vi "Get KeyValues.vi"(8 "error in (no error)":errorcluster, 11 "Frames":refnum<k21>[](array[refnum])) -> (0 "error out":errorcluster, 1 "<JSON>":string caption="<JSON>Object", 2 "Sigs":refnum<k21>[](array[refnum]), 3 "Signal Names":string[](array[string]))   [LabVIEW 2019, in "CAN.lvclass"]
uses:
  CAN.lvclass
  <vilib>/JDP Science/JSONtext/support/Format JSON Object.vi
  <resource>/objmgr/xnet.rc
  <vilib>/JDP Science/JSONtext/JSONtext.lvlib
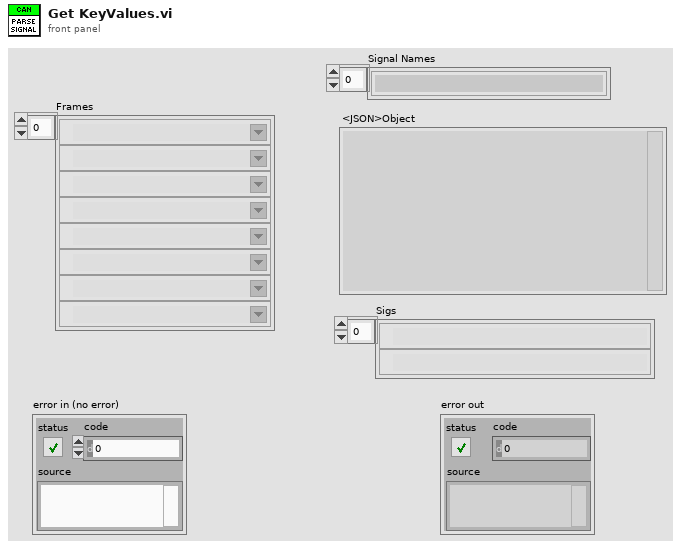
[diagram p1: front panel]
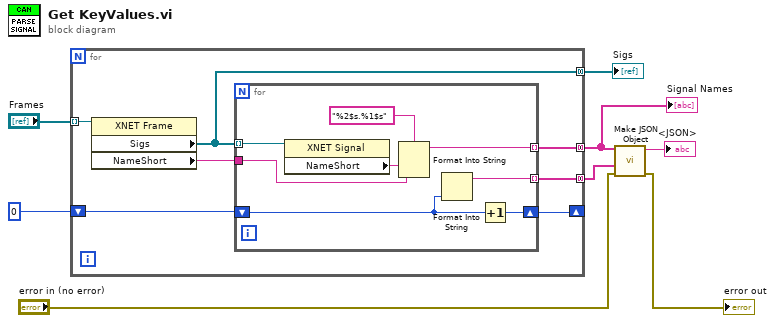
[diagram p0: block diagram]
diagram:
  n1 = for {
    tunnel: "Frames" -> [w10] mode=indexing
    shift-right: [w14] -> _
    shift-left: 0 ("Numeric") -> [w11]
    tunnel: [w13] -> w5 mode=concatenating
    tunnel: [w12] -> w4 mode=concatenating
    tunnel: [w9] -> w6 mode=concatenating
    n2 = property class="XNET Frame"(reference=w10) -> ("Sigs"=w9:refnum<k21>[], "NameShort"=w15:string)  [unwired: 1 in, 2 out]
    n3 = for {
      tunnel: w9 -> [w16] mode=indexing
      tunnel: [w17] -> w13 mode=indexing
      tunnel: [w20] -> w12 mode=indexing
      shift-right: [w18] -> w14
      shift-left: w11 -> [w19]
      tunnel: w15 -> [w22]
      n4 = property class="XNET Signal"(reference=w16) -> ("NameShort"=w23:string)  [unwired: 1 in, 2 out]
      n5 = Format Into String(format string="%2$s.%1$s", w23, w22) -> (resulting string=w17:string)  [unwired: 2 in, 1 out]
      n6 = Format Into String(w19) -> (resulting string=w20:string)  [unwired: 3 in, 1 out]
      n7 = Increment(x=w19) -> (x+1=w18:i32)
    }
  }
  "Sigs" <- w6
  "Signal Names" <- w5
  n8 = call <vilib>:"Make JSON Object.vi"("error in (no error)"="error in (no error)", "JSON Items"=w4, "Item Names"=w5) -> ("error out"=→"error out":errorcluster, "<JSON>"=→"<JSON>":string)  [unwired: 7 in]
